vi "12.vi"() -> ()   [LabVIEW 2021]
panel:
  out "Numeric":i32
  in  "#divisors":i32
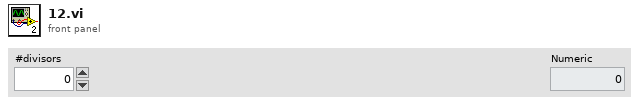
[diagram p1: front panel]
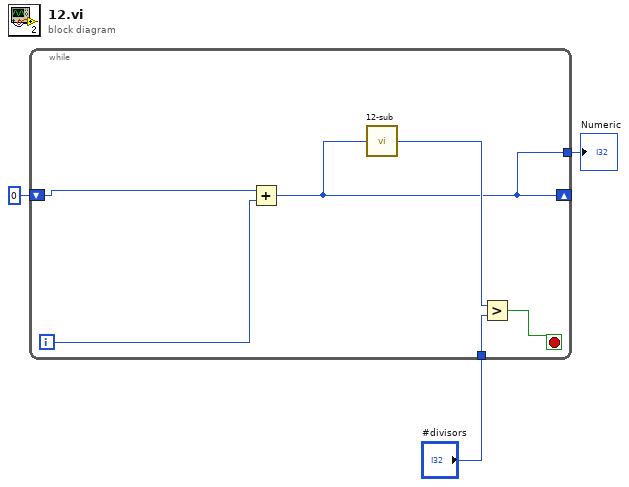
[diagram p0: block diagram]
diagram:
  n1 = while {
    shift-right: [w4] -> _
    shift-left: 0 -> [w8]
    tunnel: "#divisors" -> [w6]
    tunnel: [w4] -> w1
    i -> [w9]
    stop <- w5 stop-if-true
    n2 = Add(x=w8, y=w9) -> (x+y=w4:i32)
    n3 = call "12-sub.vi"("Numeric"=w4) -> ("size(s)"=w7:i32)
    n4 = Greater?(x=w7, y=w6) -> (0:w5:bool)
  }
  "Numeric" <- w1
